vi "CalculateCheckSum.vi"(11 "Array":u8[](array[numeric]) format="%.0b") -> (3 "checksum":u8 format="%.0b")   [LabVIEW 2016]
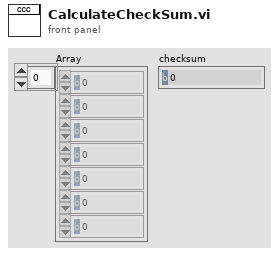
[diagram p1: front panel]
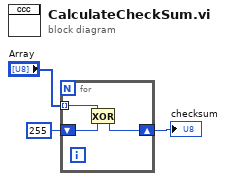
[diagram p0: block diagram]
diagram:
  n1 = for {
    tunnel: "Array" -> [w4] mode=indexing
    shift-right: [w6] -> w2
    shift-left: u8 255 -> [w5]
    n2 = Exclusive Or(1:w5, 2:w4) -> (0:w6:u8)
  }
  "checksum" <- w2
